vi "Read Header from Multiple.vi"(7 "delimiter (,)":string=",", 8 "error in":errorcluster, 10 "Name":string, 11 "Headers":refnum<class "HttpHeaders_NET.lvclass">[](array[class])) -> (0 "error out":errorcluster, 2 "Value":string, 4 "Found":bool)   [LabVIEW 2018, in "HttpClient_NET.lvlib" / "HttpHeaders_NET.lvclass"]
uses:
  HttpHeaders_NET.lvclass
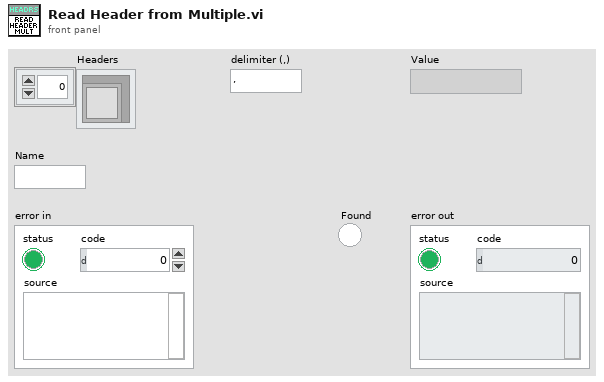
[diagram p1: front panel]
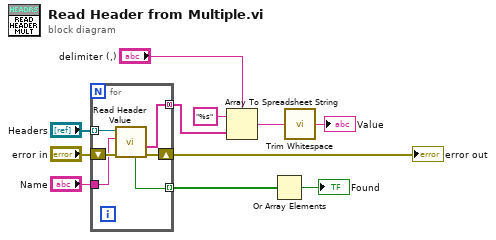
[diagram p0: block diagram]
diagram:
  n1 = for {
    tunnel: "Headers" -> [w16] mode=indexing
    tunnel: "Name" -> [w15]
    tunnel: [w14] -> w11 mode=indexing
    shift-right: [w13] -> w10
    shift-left: "error in" -> [w17]
    tunnel: [w12] -> w9 mode=concatenating
    n2 = call-dynamic "Read Header Value.vi"("error in (no error)"=w17, "Header Name"=w15, "HTTPHeaders_NET in"=w16) -> ("error out"=w13:errorcluster, "Header Value"=w12:string[], "Found"=w14:bool)  [unwired: 4 in, 2 out]
  }
  "error out" <- w10
  n3 = Array To Spreadsheet String(delimiter (Tab)="delimiter (,)", array=w9, 3:"%s" ("format string")) -> (spreadsheet string=w8:string)
  n4 = Or Array Elements(Boolean array=w11) -> (logical OR=→"Found":bool)
  n5 = call <vilib>:"Trim Whitespace.vi"("string"=w8) -> ("trimmed string"=→"Value":string)  [unwired: 1 in]
